vi "Player Info.vi"(11 "Line Dancer in":refnum<class "Swirly Vortex of Terror.lvclass">) -> (0 "Defeat Speech":string, 1 "Victory Speech":string, 2 "Name":string, 3 "Line Dancer out":refnum<class "Swirly Vortex of Terror.lvclass">)   [LabVIEW 2015, in "Swirly Vortex of Terror.lvclass"]
uses:
  Swirly Vortex of Terror.lvclass
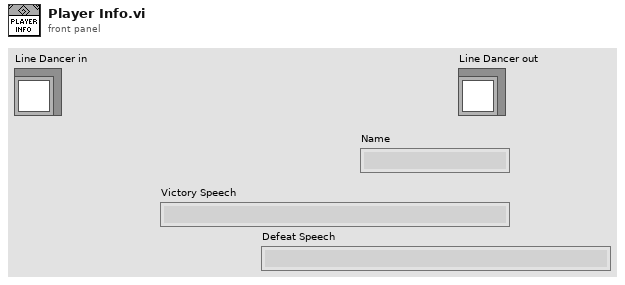
[diagram p1: front panel]
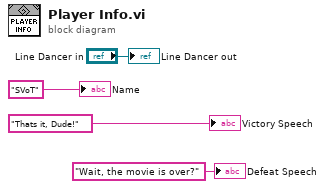
[diagram p0: block diagram]
diagram:
  "Line Dancer out" <- "Line Dancer in"
  "Name" <- "SVoT" ("Name")
  "Victory Speech" <- "Thats it, Dude!" ("Victory Speech")
  "Defeat Speech" <- "Wait, the movie is over?" ("Defeat Speech")
